vi "GT Get Axis Band.vi"(7 "pTime":i32, 8 "error in (no error)":errorcluster caption="错误输入（无错误）", 9 "pBand":i32[](array[numeric]), 10 "axis":i16, 11 "cardNum":i16) -> (0 "error out":errorcluster caption="错误输出", 1 "pBand out":i32[](array[numeric]), 3 "function return":i16, 5 "pTime out":i32)   [LabVIEW 2014, in "gts.lvlib"]
doc: "GT_API GT_GetAxisBand(short cardNum,short axis,long *pBand,long *pTime);"
uses:
  gts.lvlib
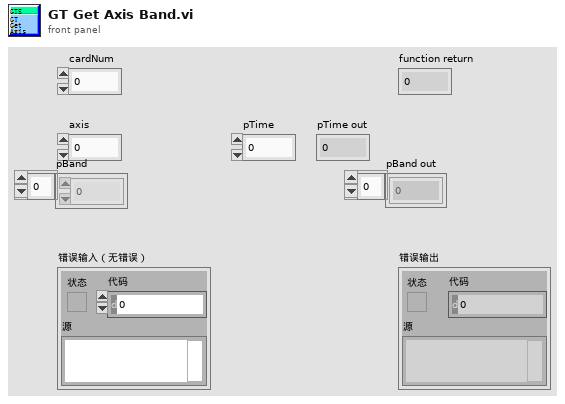
[diagram p1: front panel]
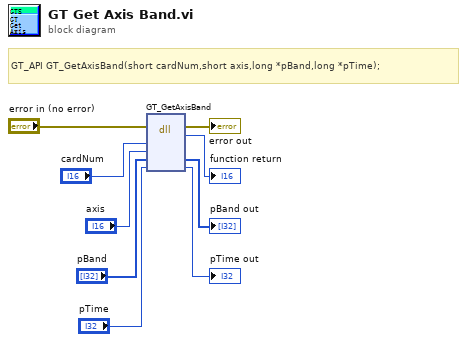
[diagram p0: block diagram]
diagram:
  # "GT_API GT_GetAxisBand(short cardNum,short axis,long *pBand,long *pTime);"
  n1 = dll-call lib="PTH2habs D固高科技资料GTS控制卡GTS卡18年上半年资料dllVC32bit\nmulti_cardgts.*" fn="GT_GetAxisBand"(error in="error in (no error)", "cardNum"="cardNum", "axis"="axis", "pBand"="pBand", "pTime"="pTime") -> (error out=→"error out":errorcluster, "返回类型"=→"function return":i16, "pBand"=→"pBand out":i32[], "pTime"=→"pTime out":i32)  [unwired: 4 in, 1 out]
